vi "Send OOB RX.vi"(8 "error in (no error)":errorcluster, 11 "CIFTemplatePlugin in":refnum<class "CIFTemplatePlugin.lvclass">) -> (0 "error out":errorcluster, 3 "CIFTemplatePlugin out":refnum<class "CIFTemplatePlugin.lvclass">)   [LabVIEW 2021, in "CIFTemplatePlugin.lvclass"]
uses:
  CIFTemplatePlugin.lvclass
  D:/dev/CIF-LVCore/src/CIFCore/Class/CIFCorePlugin.lvclass
  CIFCore/Class/CIFCorePlugin.lvclass/CIFCorePlugin.ctl
  CIFTemplatePlugin.lvclass/CIFTemplatePlugin.ctl
  OOB/OOB_Rx/Typedef/Cyclic Data.ctl
  CIFUtilities/CIFOutOfBand/CIFOutOfBand.lvclass/CIFOutOfBand.ctl
  CIFUtilities/CIFOutOfBand/Write OOB DVR.vi
  CIFUtilities/CIFOutOfBand/Utilities/Command to Bitwise Command.vi
  CIFUtilities/CIFOutOfBand/Accessors/Read Local OOB Data.vi
  CIFUtilities/CIFOutOfBand/Accessors/Write Local OOB Data.vi
  OOB/OOB_Rx/CIFTCustomOOB_Rx.lvclass
  D:/dev/CIF-LVCore/src/CIFUtilities/CIFOutOfBand/CIFOutOfBand.lvclass
  CIFCore/Class/CIFCorePlugin.lvclass
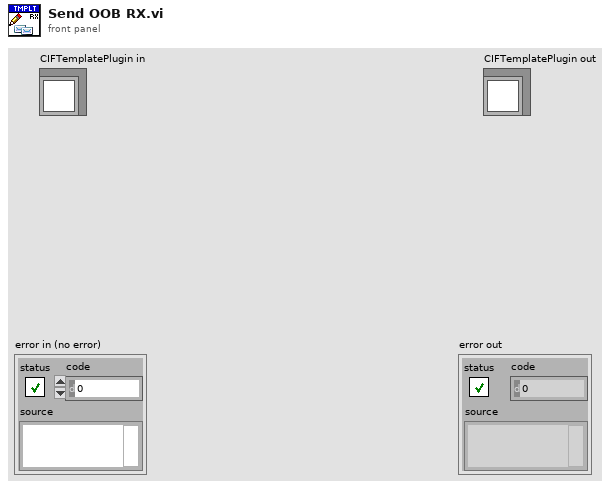
[diagram p1: front panel]
types:
  T1 = typedef "CIFTCustomOOB_Rx.lvclass/Cyclic Data.ctl" = cluster{"Numeric":i32}
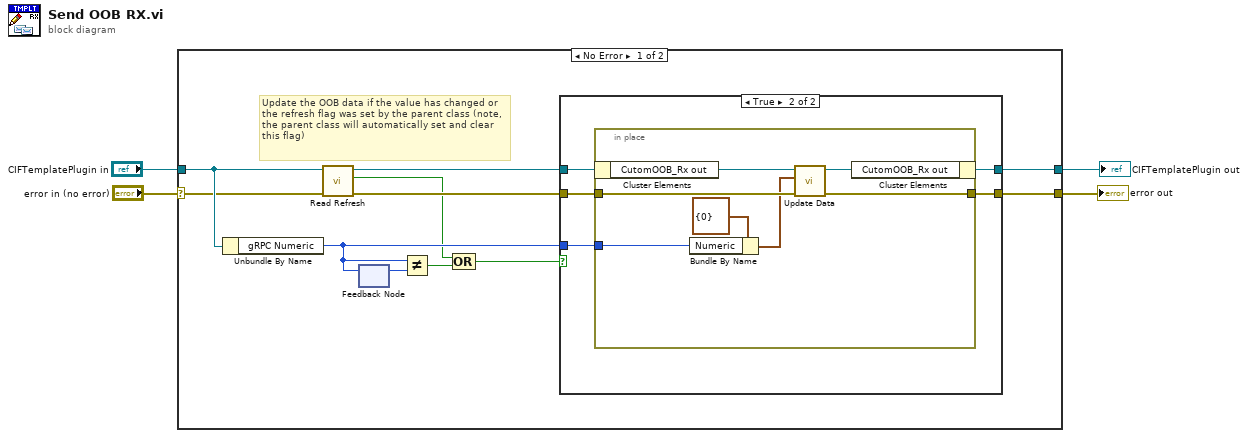
[diagram p0: block diagram]
diagram:
  n1 = case shown="No Error" "error in (no error)" {
    selector: "error in (no error)" -> [w8 w31]
    tunnel: [w10 w31] -> w3
    tunnel: [w11 w30] -> w1
    tunnel: "CIFTemplatePlugin in" -> [w9 w30]
    frame No Error {
      # "Update the OOB data if the value has changed or the refresh flag was set by the parent class (note, the parent class will automatically set and clear this flag)"
      n2 = Unbundle By Name(w9) -> ("gRPC Numeric"=w13:i32)
      n3 = call "Read Refresh.vi"("error in (no error)"=w8, "CIFCorePlugin in"=w9) -> ("error out"=w6:errorcluster, "Refresh"=w5:bool, "CIFCorePlugin out"=w7:refnum<class "CIFTemplatePlugin.lvclass">)  [unwired: 7 in]
      n4 = feedback-in #1(w13) -> ()
      n5 = feedback #1() -> (w15:i32)  [unwired: 1 in]
      n6 = Not Equal?(x=w13, y=w15) -> (x != y?=w14:bool)
      n7 = Compound Arithmetic op=OR(w5, w14) -> (w12:bool)
      n8 = case shown="True" w12 {
        tunnel: w6 -> [w16 w22]
        tunnel: w7 -> [w17 w21]
        tunnel: w13 -> [_ w20]
        tunnel: [w17 w19] -> w11
        tunnel: [w16 w18] -> w10
        frame False {
        }
        frame True {
          n9 = in-place {
            in-place-border: w22 -> [w27]
            in-place-border: [w25] -> w18
            in-place-border: w20 -> [w29]
            n10 = in-place-cluster #2(w21) -> ("CutomOOB_Rx out"=w28:refnum<class "CIFTCustomOOB_Rx.lvclass">)
            n11 = Bundle By Name(cluster=T1 {"Numeric"=0} ("Data"), "Numeric"=w29) -> (w24:T1)
            n12 = call "Update Data.vi"("error in"=w27, "Data"=w24, "CutomOOB_Rx in"=w28) -> ("error out"=w25:errorcluster, "CutomOOB_Rx out"=w26:refnum<class "CIFTCustomOOB_Rx.lvclass">)  [unwired: 7 in]
            n13 = in-place-cluster #2("CutomOOB_Rx out"=w26) -> (w19:refnum<class "CIFTemplatePlugin.lvclass">)
          }
        }
      }
    }
    frame Error {
    }
  }
  "error out" <- w3
  "CIFTemplatePlugin out" <- w1
